vi "Column Headers from SQL Query Recordset.vi"(8 "error in (no error)":errorcluster, 11 "recordset reference":T1) -> (0 "error out":errorcluster, 1 "column information":T3(array[cluster]), 2 "columns":string[](array[string]), 3 "Recordset reference Out":T1)   [LabVIEW 2010]
uses:
  <vilib>/addons/database/Auxilliary.llb/DB Tools DataTypes.ctl
  <vilib>/addons/database/Recordset.llb/Rec ObjectReference.ctl
  <vilib>/addons/database/Recordset.llb/Rec Get Recordset Properties (R).vi
  <vilib>/addons/database/Recordset.llb/Rec Get Column Properties (R).vi
  <vilib>/addons/database/NI_Database_API.lvlib
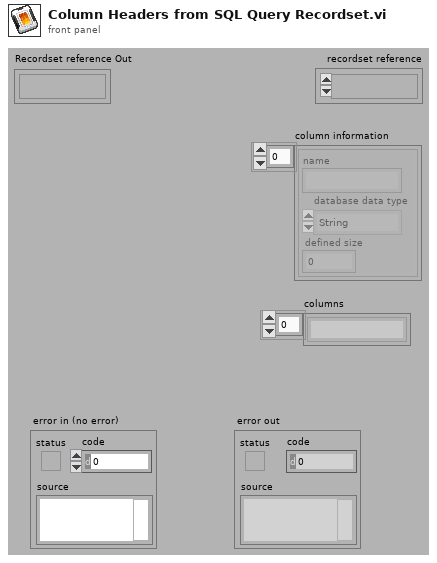
[diagram p1: front panel]
types:
  T1 = typedef "NI_Database_API.lvlib/Rec ObjectReference.ctl" = refnum<k1>
  T2 = typedef "NI_Database_API.lvlib/DB Tools DataTypes.ctl" = enum16{"String", "Long (I32)", "Single (SGL)", "Double (DBL)", "Date/Time", "Binary"}
  T3 = cluster{"name":string, "database data type":T2, "defined size":i32}[]
  T4 = cluster{"name":string, "database data type":enum16{"String", "Long (I32)", "Single (SGL)", "Double (DBL)", "Date/Time", "Binary"}, "defined size":i32}[]
  T5 = typedef "NI_Database_API.lvlib/Rec Properties.ctl" = cluster{"column count":i32, "record index":i32, "record count":i32, "bof?":bool, "eof?":bool, "cursor type":T6, "cache size":i32, "state":enum16{"closed", "open"}}
  T6 = typedef "NI_Database_API.lvlib/DB Tools Cursor Type.ctl" = enum16{"forward-only", "keyset", "dynamic", "static"}
  T7 = typedef "NI_Database_API.lvlib/Rec Column Properties.ctl" = cluster{"name":string, "database data type":T2, "defined size":i32, "actual size":i32}
  T8 = cluster{"name":string, "database data type":T2, "defined size":i32}
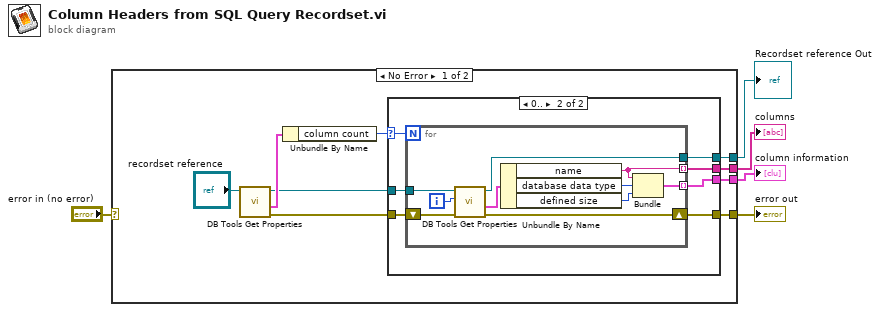
[diagram p0: block diagram]
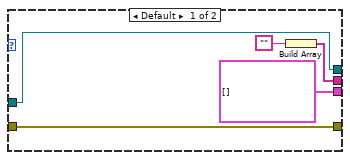
[diagram p2: hidden frame]
diagram:
  n1 = case shown="No Error" "error in (no error)" {
    selector: "error in (no error)" -> [_ w37]
    tunnel: [w7 _] -> w1
    tunnel: [w11 _] -> w2
    tunnel: [w10 _] -> w3
    tunnel: [w6 w37] -> w4
    frame No Error {
      n2 = call-poly <vilib>:"DB Tools Get Properties.vi"("recordset reference"="recordset reference") -> ("error out"=w12:errorcluster, "recordset properties"=w14:T5, "recordset reference out"=w13:T1)  [unwired: 4 in]
      n3 = Unbundle By Name(w14) -> ("column count"=w9:i32)
      n4 = case shown="0.." w9 {
        selector: w9 -> [_ w20]
        tunnel: w13 -> [w19 w26]
        tunnel: w12 -> [w18 w25]
        tunnel: [w18 w24] -> w6
        tunnel: [w19 w23] -> w7
        tunnel: [T4 [] w22] -> w11
        tunnel: [w16 w21] -> w10
        frame Default {
          n5 = Build Array("") -> (w16:string[])
        }
        frame 0.. {
          n6 = for {
            N: w20 -> [_]
            tunnel: w26 -> [w35]
            shift-right: [w30] -> w24
            shift-left: w25 -> [w36]
            tunnel: [w31] -> w22 mode=indexing
            tunnel: [w29] -> w23
            tunnel: [w27] -> w21 mode=indexing
            i -> [w34]
            n7 = call-poly <vilib>:"DB Tools Get Properties.vi"("error in (no error)"=w36, "column index"=w34, "recordset reference"=w35) -> ("error out"=w30:errorcluster, "column properties"=w33:T7, "recordset reference out"=w29:T1)  [unwired: 2 in]
            n8 = Unbundle By Name(w33) -> ("name"=w27:string, "database data type"=w32:T2, "defined size"=w28:i32)
            n9 = Bundle("name"=w27, "database data type"=w32, "defined size"=w28) -> (w31:T8)  [unwired: 1 in]
          }
        }
      }
    }
    frame Error {
    }
  }
  "error out" <- w4
  "column information" <- w2
  "columns" <- w3
  "Recordset reference Out" <- w1
